vi "Save.vi"(8 "error in (no error)":errorcluster, 9 "overwrite file (True)":bool=TRUE, 10 "XML file path":path, 11 "DOM document in":refnum<k20>) -> (0 "error out":errorcluster, 2 "XML file path out":path, 3 "DOM document out":refnum<k20>)   [LabVIEW 2017, in "NI_XML.lvlib"]
doc: "Saves an XML document."
uses:
  <vilib>/xml/NI_XML.lvlib
  <resource>/objmgr/DOMUserDefRef.rc
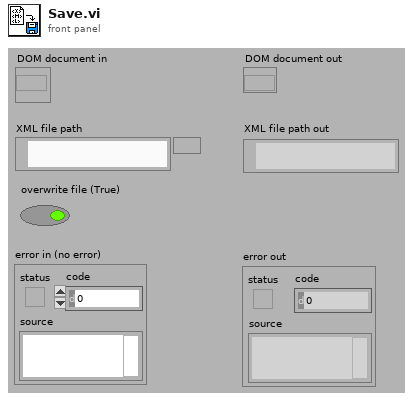
[diagram p1: front panel]
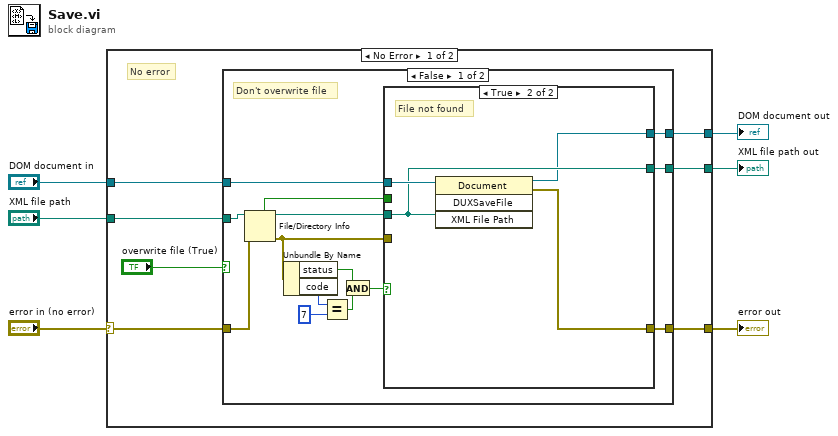
[diagram p0: block diagram]
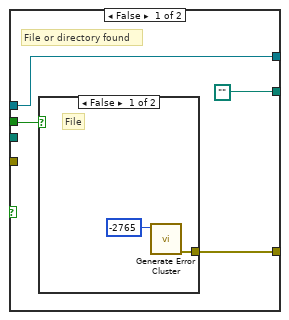
[diagram p2: hidden frame]
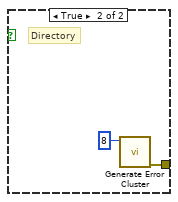
[diagram p3: hidden frame]
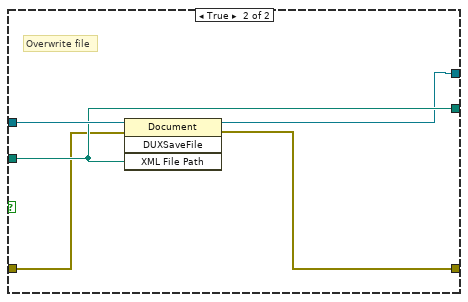
[diagram p4: hidden frame]
diagram:
  n1 = case shown="No Error" "error in (no error)" {
    selector: "error in (no error)" -> [w7 w47]
    tunnel: [w12 w47] -> w5
    tunnel: [w11 w45] -> w4
    tunnel: "DOM document in" -> [w10 w46]
    tunnel: "XML file path" -> [w9 w45]
    tunnel: [w8 w46] -> w1
    frame No Error {
      # "No error"
      n2 = case shown="False" "overwrite file (True)" {
        tunnel: w9 -> [w27 w42]
        tunnel: w10 -> [w19 w44]
        tunnel: [w18 w43] -> w12
        tunnel: [w17 w42] -> w11
        tunnel: [w16 w41] -> w8
        tunnel: w7 -> [w15 w40]
        frame False {
          # "Don't overwrite file"
          n3 = File/Directory Info(path=w27, error in=w15) -> (path out=w26:path, directory=w25:bool, error out=w14:errorcluster)  [unwired: 4 out]
          n4 = Unbundle By Name(w14) -> ("status"=w21:bool, "code"=w24:i32)
          n5 = Equal?(x=w24, y=7) -> (x = y?=w20:bool)
          n6 = And(x=w21, y=w20) -> (x .and. y?=w22:bool)
          n7 = case shown="True" w22 {
            tunnel: w26 -> [_ w37]
            tunnel: w25 -> [w31 _]
            tunnel: w19 -> [w28 w39]
            tunnel: [w30 w38] -> w18
            tunnel: [path "" w37] -> w17
            tunnel: [w28 w36] -> w16
            tunnel: w14 -> [_ _]
            frame False {
              # "File or directory found"
              n8 = case shown="False" w31 {
                tunnel: [w32 w34] -> w30
                frame False {
                  # "File"
                  n9 = call <vilib>:"Generate Error Cluster.vi"("Code"=-2765) -> ("error out"=w32:errorcluster)  [unwired: 2 in, 8 out]
                }
                frame True {
                  # "Directory"
                  n10 = call <vilib>:"Generate Error Cluster.vi"("Code"=8) -> ("error out"=w34:errorcluster)  [unwired: 2 in, 8 out]
                }
              }
            }
            frame True {
              # "File not found"
              n11 = invoke class="Document" method="DUXSaveFile"(reference=w39, "XML File Path"=w37) -> (reference out=w36:refnum<k20>, error out=w38:errorcluster)  [unwired: 2 in, 2 out]
            }
          }
        }
        frame True {
          # "Overwrite file"
          n12 = invoke class="Document" method="DUXSaveFile"(reference=w44, error in=w40, "XML File Path"=w42) -> (reference out=w41:refnum<k20>, error out=w43:errorcluster)  [unwired: 1 in, 2 out]
        }
      }
    }
    frame Error {
      # "Error"
    }
  }
  "error out" <- w5
  "XML file path out" <- w4
  "DOM document out" <- w1
